vi "AccelnetVelScale.vi"(1 "Acelnet eCAT vel":i32) -> (0 "Shaft vel (rad/s)":dbl)   [LabVIEW 2018]
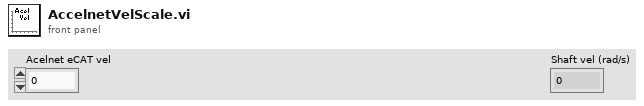
[diagram p1: front panel]
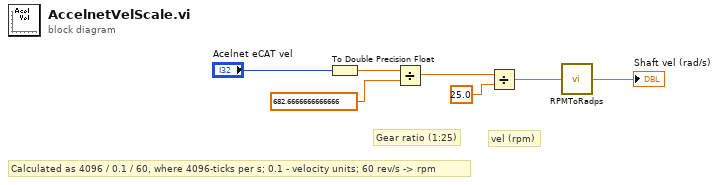
[diagram p0: block diagram]
diagram:
  # "vel (rpm)"
  # "Calculated as 4096 / 0.1 / 60, where 4096-ticks per s; 0.1 - velocity units; 60 rev/s -> rpm"
  # "Gear ratio (1:25)"
  n1 = To Double Precision Float(number="Acelnet eCAT vel") -> (double precision float=w6:dbl)
  n2 = Divide(x=w6, y=682.6666666666666) -> (x/y=w4:dbl)
  n3 = Divide(x=w4, y=25.0) -> (x/y=w2:dbl)
  n4 = call "RPMToRadps.vi"("rpm"=w2) -> ("rad/s"=→"Shaft vel (rad/s)":dbl)
